vi "cblas dasum.vi"(5 "n":i32=-1, 7 "incx":i32=1, 11 "x":dbl[](array[numeric])) -> (0 "error":i32, 3 "dasum":dbl)   [LabVIEW 2018, in "NI_AALBLAS.lvlib"]
doc: "Calculates the sum of the absolute values of elements in <B>X</B> with indexes that are multiples of <B>incX</B>. The data type you wire to the <B>X</B> input determines the polymorphic instance to use."
uses:
  NI_AALBLAS.lvlib
  <resource>/lvblas.dll
panel:
  # "double cblas_dasum(n, *x, incx)"
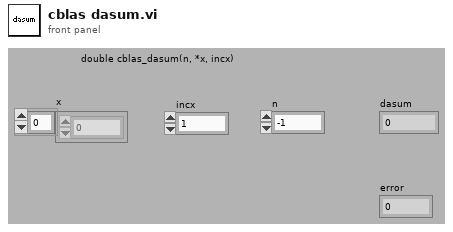
[diagram p1: front panel]
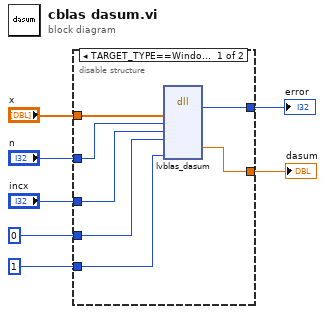
[diagram p0: block diagram]
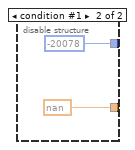
[diagram p2: hidden frame]
diagram:
  n1 = disable-structure shown="TARGET_TYPE==Windows||TARGET_TYPE==Unix||TARGET_TYPE==Mac||TARGET_TYPE==RT" {
    disable-tunnel: "x" -> [w13 _]
    disable-tunnel: "n" -> [w12 _]
    disable-tunnel: "incx" -> [w11 _]
    disable-tunnel: [w10 nan] -> w4
    disable-tunnel: [w14 -20078] -> w3
    disable-tunnel: 0 -> [w9 _]
    disable-tunnel: 1 -> [w8 _]
    frame condition #0 (active) {
      n2 = dll-call lib="C:/Program Files (x86)/National Instruments/LabVIEW 2018/resource/lvblas.*" fn="lvblas_dasum" ("LVBLAS.dll:BLASVectorSumH")("X"=w13, "N"=w12, "IncX"=w11, "startX"=w9, "check"=w8) -> ("error"=w14:i32, "dasum"=w10:dbl)  [unwired: 8 in, 3 out]
    }
    frame condition #1 {
    }
  }
  "dasum" <- w4
  "error" <- w3
